vi "Example Kafka Read Events Data.vi"() -> ()   [LabVIEW 2019]
doc: "This example demonstrates how to read measured data, text and timestamps from a .tdms file using the TDMS API."
uses:
  support/_readType.ctl
panel:
  out "Property Values":variant[][](array[variant])
  out "Property Names":string[][](array[string])
  out "Measured Data":waveform(dbl)[](graph)
  # "Overview: Demonstrates the use of the TDMS Read function to read measured data, text and timestamps from an existing .tdms file.\nInstructions:\n1. Make sure you have already run TDMS Write Events Data.vi.\n2. Run this VI.\n3. Delete the .tdms file (located at [LabVIEW Data]\\Example Events Data.tdms) when you are done."
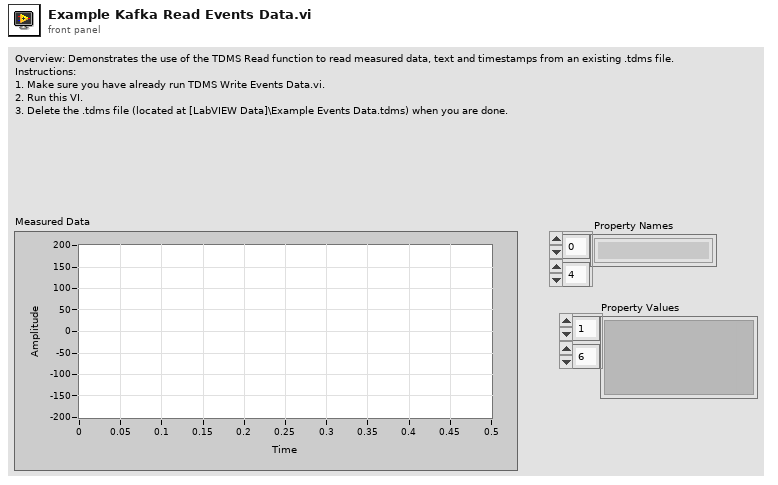
[diagram p1: front panel]
types:
  T1 = typedef "_readType.ctl" = enum16{"All", "Real-time", "Start Offset"}
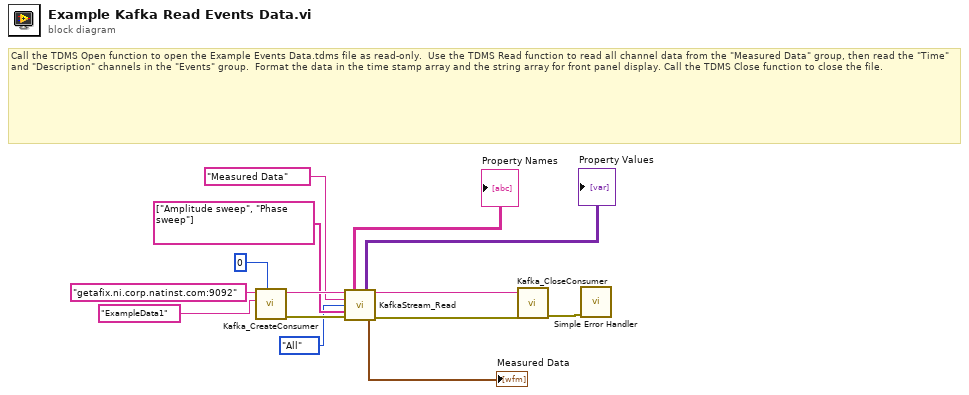
[diagram p0: block diagram]
diagram:
  # "Call the TDMS Open function to open the Example Events Data.tdms file as read-only.  Use the TDMS Read function to read all channel data from the \"Measured Data\" group, then read the \"Time\" and \"Description\" channels in the \"Events\" group.  Format the data in the time stamp array and the string array for front panel display. Call the TDMS Close function to close the file."
  n1 = call "Kafka_CreateConsumer.vi"("Partition"=0, "Topic"="ExampleData1", "Kafka Broker"="getafix.ni.corp.natinst.com:9092") -> ("error out"=w11:errorcluster, "Consumer Handle"=w10:string)  [unwired: 7 in]
  n2 = call "KafkaStream_Read.vi"("Consumer Handle"=w10, "Group Name"="Measured Data" ("group name"), "Read Type"=_readType."All", "Channel Names"=string[] ["Amplitude sweep", "Phase sweep"] ("channel names"), "error in (no error)"=w11) -> ("Property Names"=→"Property Names":string[][], "Property Values"=→"Property Values":variant[][], "Consumer Handle Out"=w6:string, "Waveforms"=→"Measured Data":waveform(dbl)[], "error out"=w5:errorcluster)  [unwired: 4 in, 2 out]
  n3 = call "Kafka_CloseConsumer.vi"("error in (no error)"=w5, "Consumer Handle"=w6) -> ("error out"=w4:errorcluster)  [unwired: 8 in, 1 out]
  n4 = call <vilib>:"Simple Error Handler.vi"("error in (no error)"=w4) -> ()  [unwired: 2 in, 7 out]
